vi "LIBUMP_ARG_UNDEF.vi"(8 "Error In":errorcluster) -> (0 "Error Out":errorcluster, 3 "LIBUMP_ARG_UNDEF":i32)   [LabVIEW 2016, in "OSB_uMp_library.lvlib"]
doc: "Constant that can be used as an argument to pass to functions when a null is required but 0 would be a valid value (i.e. 0 would not represent null)."
uses:
  OSB_uMp_library.lvlib
panel:
  # "By Stuart Box at OxSyBio Ltd, 2017\n\nThis software is provided WITHOUT ANY WARRANTY; without even the implied warranty of MERCHANTABILITY or FITNESS FOR A PARTICULAR PURPOSE.\n\ninfo@oxsybio.com\n\nOxSyBio Ltd, The Walbrook Building, 25 Walbrook, London, EC4N 8AF"
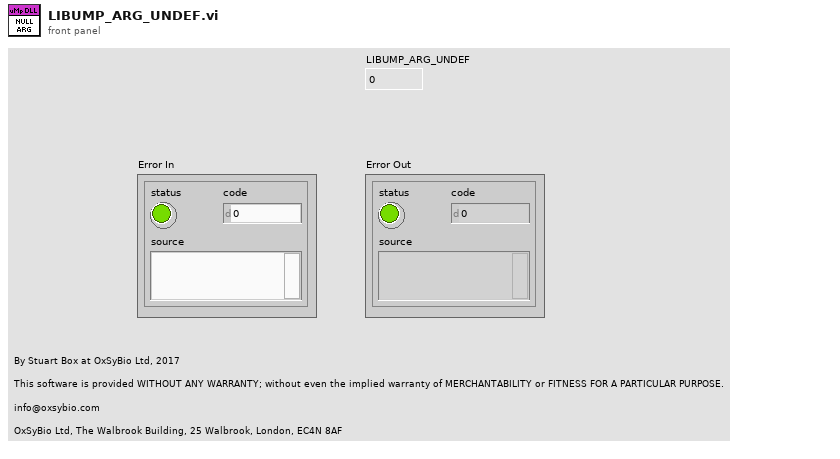
[diagram p1: front panel]
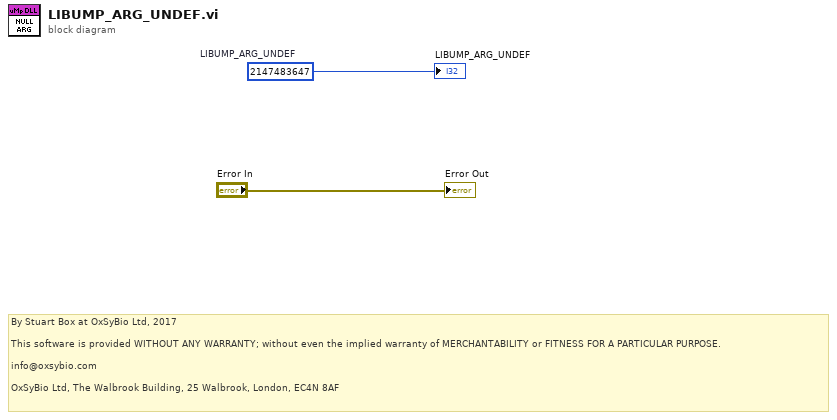
[diagram p0: block diagram]
diagram:
  w1 = 2147483647  # LIBUMP_ARG_UNDEF
  # "By Stuart Box at OxSyBio Ltd, 2017\n\nThis software is provided WITHOUT ANY WARRANTY; without even the implied warranty of MERCHANTABILITY or FITNESS FOR A PARTICULAR PURPOSE.\n\ninfo@oxsybio.com\n\nOxSyBio Ltd, The Walbrook Building, 25 Walbrook, London, EC4N 8AF"
  "Error Out" <- "Error In"
  "LIBUMP_ARG_UNDEF" <- w1
